vi "ControlSystem.vi"(0 "File Path":path[](array[path]), 5 "Ignition":bool, 7 "Deadman":bool, 9 "Dry Test Run":bool, 11 "Maintain Pressure":bool, 12 "Sensor Values":dbl[](array[numeric])) -> (1 "PT1E":bool, 2 "PT2E":bool, 3 "PT3E":bool, 4 "FM1E":bool, 6 "FM2E":bool, 8 "Abort":bool, 10 "DTR Done":bool, 13 "TC1E":bool, 14 "TC2E":bool, 15 "Solenoid Outputs":bool[](array[boolean]))   [LabVIEW 2021]
uses:
  <vilib>/Utility/file.llb/Read Delimited Spreadsheet (string).vi
panel:
  out "error out":errorcluster
  in  "error in":errorcluster
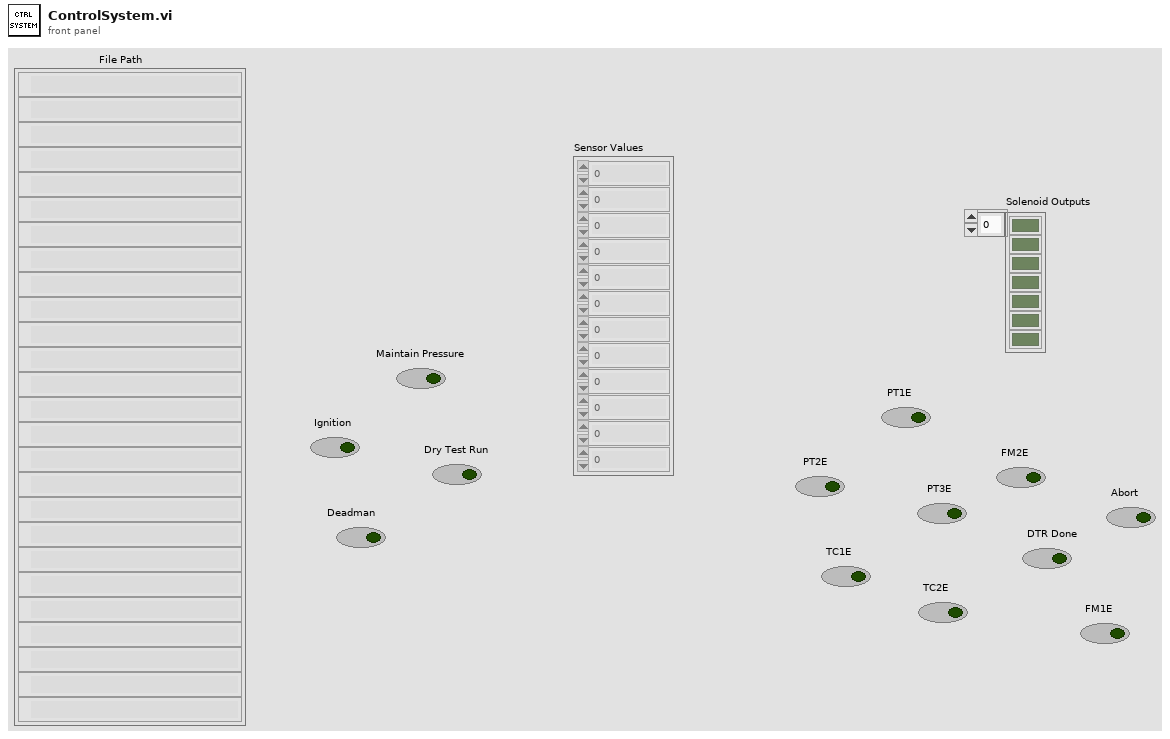
[diagram p1: front panel]
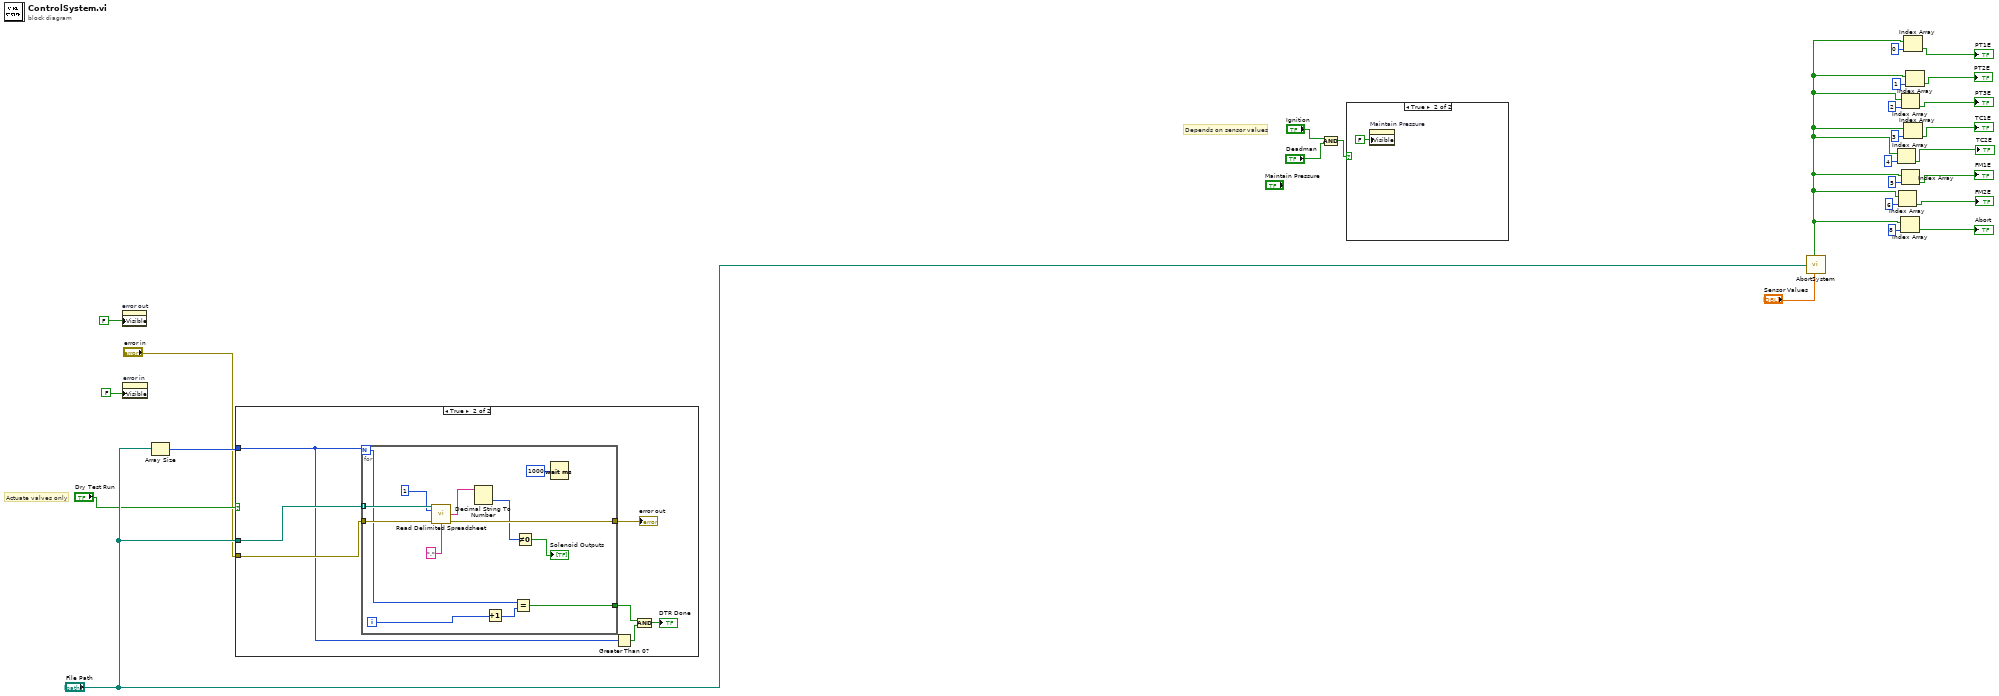
[diagram p0: block diagram]
diagram:
  # "Actuate valves only"
  # "Depends on sensor values"
  n1 = property on="error out" class="Clust (strict)"("Visible"=FALSE) -> ()  [unwired: 2 in, 2 out]
  n2 = property on="error in" class="Clust (strict)"("Visible"=FALSE) -> ()  [unwired: 2 in, 2 out]
  n3 = Array Size(array="File Path") -> (size(s)=w2:i32)
  n4 = case shown="True" "Dry Test Run" {
    tunnel: w2 -> [_ w29]
    tunnel: "File Path" -> [_ w32]
    tunnel: "error in" -> [_ w33]
    frame False {
    }
    frame True {
      n5 = for {
        N: w29 -> [w38]
        tunnel: w32 -> [w47] mode=indexing
        tunnel: w33 -> [w44]
        tunnel: [w43] -> w34
        tunnel: [w37] -> w31
        i -> [w39]
        n6 = call-poly <vilib>:"Read Delimited Spreadsheet.vi"("file path (dialog if empty)"=w47, "number of rows (all:-1)"=1, "error in (no error)"=w44, "delimiter (\\t)"="," ("delimiter (\\t)")) -> ("first row"=w42:string[], "error out"=w43:errorcluster)  [unwired: 6 in, 4 out]
        n7 = Decimal String To Number(string=w42) -> (number=w41:i32[])  [unwired: 2 in, 1 out]
        n8 = Increment(x=w39) -> (x+1=w40:i32)
        n9 = Equal?(x=w38, y=w40) -> (x = y?=w37:bool)
        n10 = Not Equal To 0?(x=w41) -> (x != 0?=→"Solenoid Outputs":bool[])
        n11 = Wait (ms)(milliseconds to wait=u32 1000) -> ()  [unwired: 1 out]
      }
      "error out" <- w34
      n12 = Greater Than 0?(x=w29) -> (x > 0?=w30:bool)
      n13 = And(x=w31, y=w30) -> (x .and. y?=→"DTR Done":bool)
    }
  }
  n14 = And(x="Ignition", y="Deadman") -> (x .and. y?=w7:bool)
  n15 = case shown="True" w7 {
    frame False {
    }
    frame True {
      n16 = property on="Maintain Pressure" class="Bool (strict)"("Visible"=FALSE) -> ()  [unwired: 2 in, 2 out]
    }
  }
  n17 = call "AbortSystem.vi"("File Path"="File Path", "Sensor Readings"="Sensor Values") -> ("Abort Status"=w8:bool[])  [unwired: 2 in, 1 out]
  n18 = Index Array(array=w8, index=4) -> (element=→"TC2E":bool)
  n19 = Index Array(array=w8, index=6) -> (element=→"FM2E":bool)
  n20 = Index Array(array=w8, index=8) -> (element=→"Abort":bool)
  n21 = Index Array(array=w8, index=2) -> (element=→"PT3E":bool)
  n22 = Index Array(array=w8, index=5) -> (element=→"FM1E":bool)
  n23 = Index Array(array=w8, index=0) -> (element=→"PT1E":bool)
  n24 = Index Array(array=w8, index=3) -> (element=→"TC1E":bool)
  n25 = Index Array(array=w8, index=1) -> (element=→"PT2E":bool)
